vi "Stop button.vi"(8 "error in (no error)":errorcluster, 11 "VISA resource name":refnum<visa-resource-name>) -> (0 "error out":errorcluster, 3 "VISA resource name out":refnum<visa-resource-name>)   [LabVIEW 2009, in "SR400.lvlib"]
doc: "Sending the CH command has the same effect as\npressing the STOP key. The CH command may be\nsent at any time. If recieved while scanning, the\nscan will pause. If received while paused, the\ncounters will reset. If the DWELL TIME is\nEXTERNAL, the CH command may be used to\nterminate count periods."
uses:
  SR400.lvlib
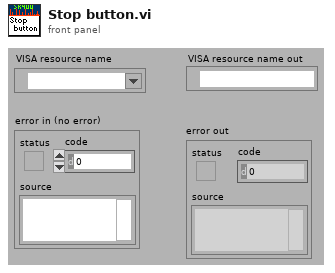
[diagram p1: front panel]
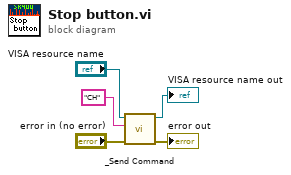
[diagram p0: block diagram]
diagram:
  n1 = call "_Send Command.vi"("error in (no error)"="error in (no error)", "Command"="CH" ("command"), "VISA resource name"="VISA resource name") -> ("error out"=→"error out":errorcluster, "VISA resource name out"=→"VISA resource name out":refnum<visa-resource-name>)  [unwired: 1 in, 6 out]
